vi "mixture_enthalpy_quality.vi"(4 "Dev Section Pressure [Pa]":dbl, 5 "Separator Temp [C]":dbl, 6 "Liquid Inlet Temp [C]":dbl, 7 "Vapor Flow Rate [g/s]":dbl, 8 "Liquid Flow Rate [g/s]":dbl) -> (0 "Quality [-]":dbl, 1 "mixture enthalpy":dbl, 2 "h_v_corr":dbl, 3 "h_l_corr":dbl)   [LabVIEW 2015]
uses:
  <vilib>/express/express arith-compare/Formula/XNode/ExpressFormulaBlockNode.xnode
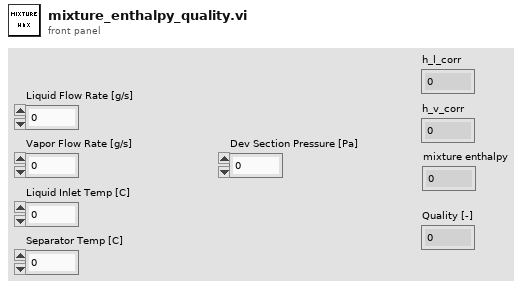
[diagram p1: front panel]
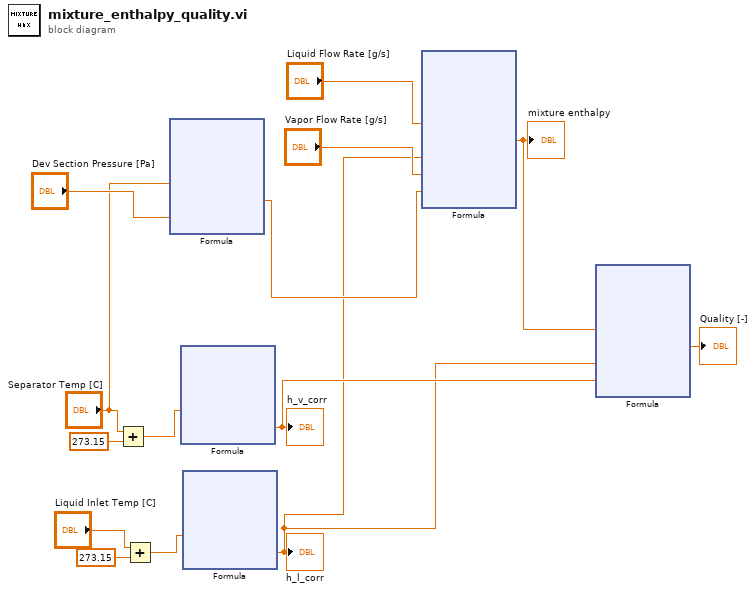
[diagram p0: block diagram]
diagram:
  n1 = Add(x="Separator Temp [C]", y=273.15) -> (x+y=w1:dbl)
  n2 = Add(x="Liquid Inlet Temp [C]", y=273.15) -> (x+y=w5:dbl)
  n3 = xnode "Formula"("T_v"="Separator Temp [C]", "P_v"="Dev Section Pressure [Pa]") -> ("Result"=w12:dbl)  [unwired: 1 in, 1 out]
  n4 = xnode "Formula"("T"=w1) -> ("Result"=w9:dbl)  [unwired: 1 in, 1 out]
  "h_v_corr" <- w9
  n5 = xnode "Formula"("T"=w5) -> ("Result"=w8:dbl)  [unwired: 1 in, 1 out]
  "h_l_corr" <- w8
  n6 = xnode "Formula"("m_dot_l"="Liquid Flow Rate [g/s]", "h_l"=w8, "m_dot_v"="Vapor Flow Rate [g/s]", "h_v"=w12) -> ("Result"=w10:dbl)  [unwired: 1 in, 1 out]
  "mixture enthalpy" <- w10
  n7 = xnode "Formula"("h_mix"=w10, "h_l"=w8, "h_v"=w9) -> ("Result"=→"Quality [-]":dbl)  [unwired: 1 in, 1 out]
